vi "Sub_Build_Variable_Header_Publish.vi"(8 "error in (no error)":errorcluster, 10 "Topic Name":string="Topic") -> (0 "error out":errorcluster, 2 "Variable Header":u8[](array[numeric]) format="%x")   [LabVIEW 2013, in "IOTFoundation.lvlib"]
uses:
  IOTFoundation.lvlib
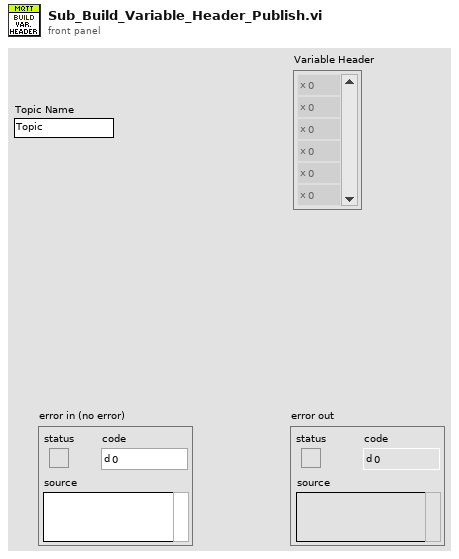
[diagram p1: front panel]
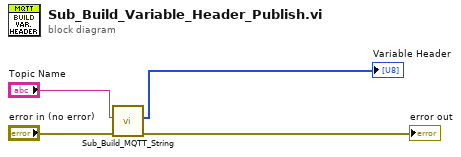
[diagram p0: block diagram]
diagram:
  n1 = call "Sub_Build_MQTT_String.vi"("error in (no error)"="error in (no error)", "String to be encoded"="Topic Name") -> ("error out"=→"error out":errorcluster, "UTF8 Byte Array"=→"Variable Header":u8[])  [unwired: 8 in]
